vi "Perform Step.vi"(8 "error in (no error)":errorcluster, 11 "Wait Action in":refnum<class "Wait Action.lvclass">) -> (0 "error out":errorcluster, 2 "Result":T1, 3 "Wait Action out":refnum<class "Wait Action.lvclass">)   [LabVIEW 2020, in "MacroAssert.lvlib" / "Wait Action.lvclass"]
uses:
  Wait Action.lvclass
  Wait Action.lvclass/Wait Action.ctl
  MacroAssert.lvlib
  CTLs/FGV Actions.ctl
  CTLs/Report Data.ctl
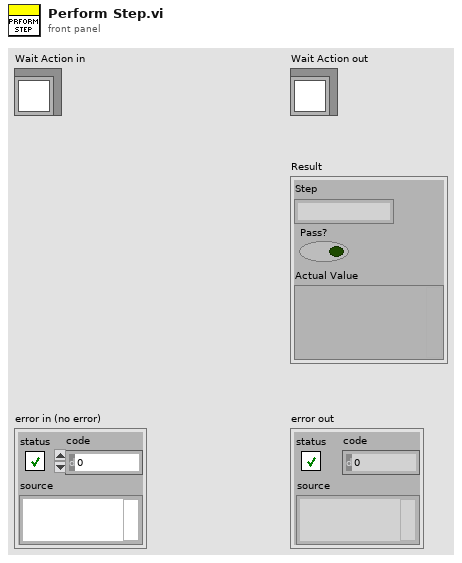
[diagram p1: front panel]
types:
  T1 = typedef "MacroAssert.lvlib/Report Data.ctl" = cluster{"Step":string, "Pass?":bool, "Actual Value":variant}
  T2 = typedef "MacroAssert.lvlib/FGV Actions.ctl" = enum16{"Read", "Write"}
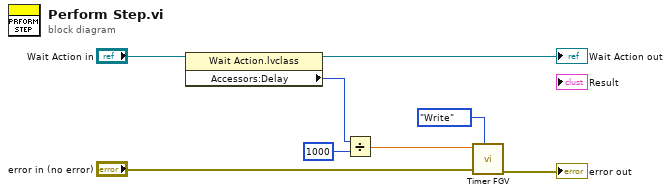
[diagram p0: block diagram]
diagram:
  n1 = property class="Wait Action.lvclass"(reference="Wait Action in") -> (reference out=→"Wait Action out":refnum<class "Wait Action.lvclass">, "Accessors:Delay"=w1:i32)  [unwired: 1 in, 1 out]
  n2 = Divide(x=w1, y=1000) -> (x/y=w4:dbl)
  n3 = call "Timer FGV.vi"("Mode"=FGV_Actions."Write", "error in (no error)"="error in (no error)", "Timer Value (s)"=w4) -> ("error out"=→"error out":errorcluster)  [unwired: 6 in, 2 out]
